vi "niTuner Get Cal (multi).vi"(8 "error in":errorcluster, 9 "correct for attenuation":bool=TRUE, 11 "taskID in":i32 format="%.0x") -> (0 "error out":errorcluster, 2 "calibrations":T1(array[cluster]) {"array" format="%.2f"; "f2" format="%.2f"; "f1" format="%.2f"}, 3 "taskID out":i32 format="%.0x")   [LabVIEW 2011]
doc: "This polymorph returns calibration information for multiple frequency entries in the scan list. Each frequency entry returns an RF calibration coefficient, an IF calibration coefficient, and (if include attenuation is set to TRUE) a total attenuation calibration coefficient."
uses:
  nipxi5600u.dll
  nidaq32.dll
panel:
  out "RF tuned frequencies":dbl[](graph)
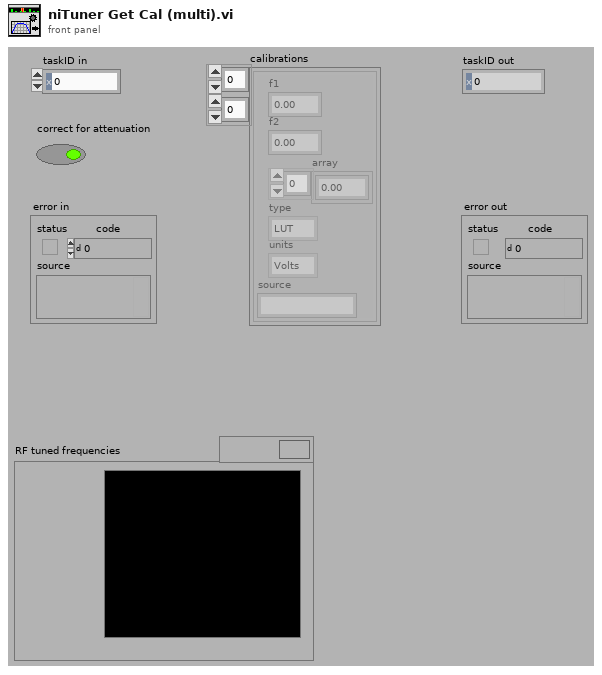
[diagram p1: front panel]
types:
  T1 = cluster{"f1":dbl, "f2":dbl, "array":sgl[], "type":enum16{"LUT", "polynomial"}, "units":enum16{"Volts", "Watts", "dBm", "dBW", "dBV", "dBmV", "dBuV"}, "source":string}[][]
  T2 = cluster{"f1":dbl, "f2":dbl, "array":sgl[], "type":enum16{"LUT", "polynomial"}, "units":enum16{"Volts", "Watts", "dBm", "dBW", "dBV", "dBmV", "dBuV"}, "source":string}
  T3 = cluster{"f1":dbl, "f2":dbl, "array":sgl[], "type":enum16{"LUT", "polynomial"}, "units":enum16{"Volts", "Watts", "dBm", "dBW", "dBV", "dBmV", "dBuV"}, "source":string}[]
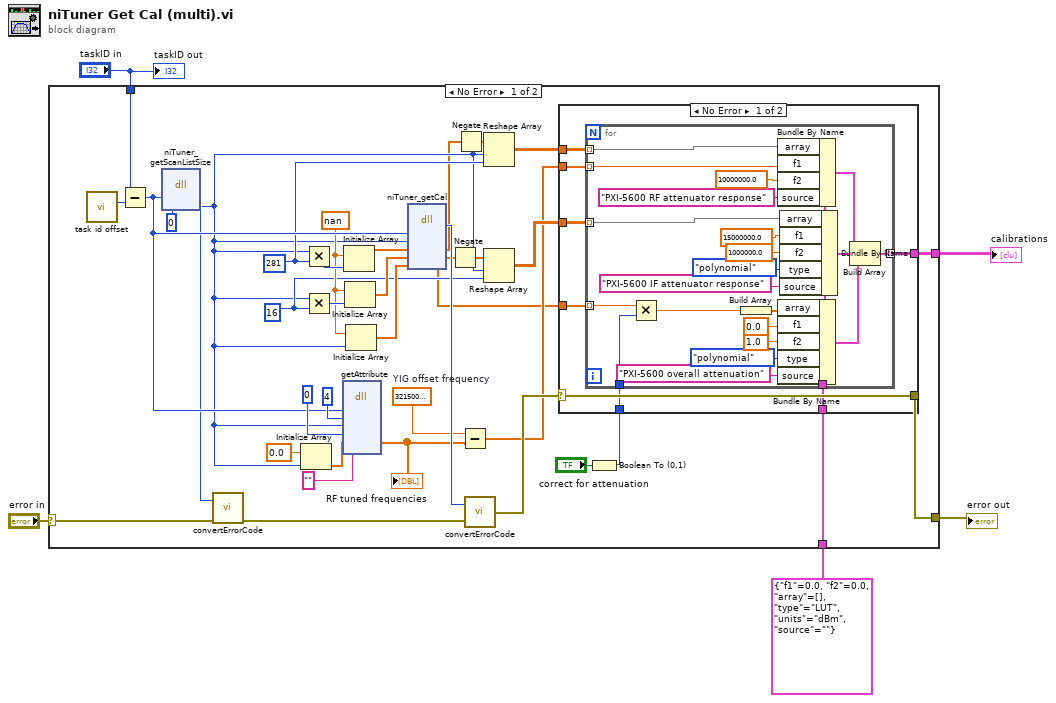
[diagram p0: block diagram]
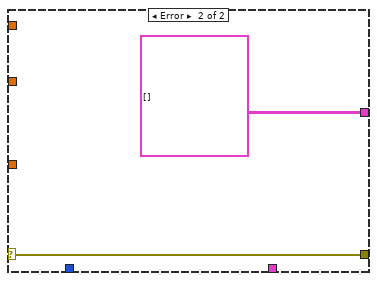
[diagram p2: hidden frame]
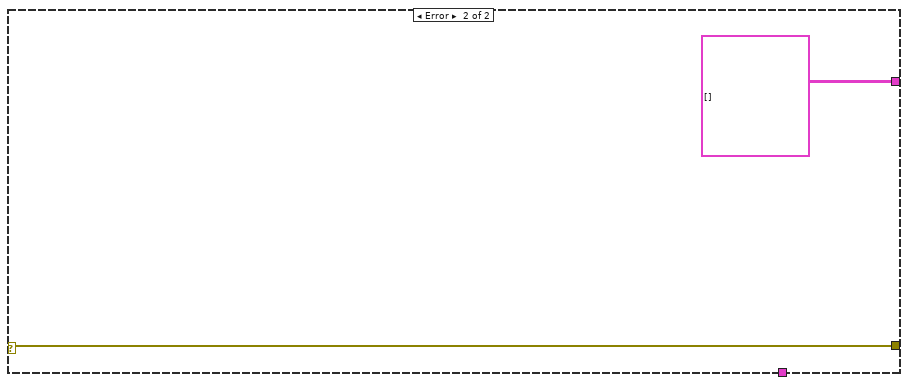
[diagram p3: hidden frame]
diagram:
  n1 = case shown="No Error" "error in" {
    selector: "error in" -> [w23 w77]
    tunnel: T2 {"f1"=0.0, "f2"=0.0, "array"=[], "type"=enum."LUT", "units"=enum."dBm", "source"=""} -> [w41 _]
    tunnel: [w40 w77] -> w3
    tunnel: "taskID in" -> [w39 _]
    tunnel: [w14 T1 []] -> w1
    frame No Error {
      w16 = 3215000000.0  # YIG offset frequency
      w27 = nan ("Element Data")
      w19 = u32 16
      w20 = u32 281
      n2 = call <instrlib>:"task id offset.vi"() -> ("taskID offset"=w43:i32)
      n3 = Subtract(x=w39, y=w43) -> (x-y=w31:i32)
      n4 = dll-call lib="nipxi5600u.dll" fn="niTuner_getScanListSize"("taskID"=w31, "scanListSize"=u32 0) -> (w24:i32, "scanListSize"=w11:u32)  [unwired: 4 in, 2 out]
      n5 = call <instrlib>:"convertErrorCode.vi"("error in"=w23, "error code"=w24) -> ("error out"=w22:errorcluster)
      n6 = Initialize Array(0.0 ("Element Data"), w11) -> (w36:dbl[])
      n7 = Multiply(x=w11, y=w20) -> (x*y=w29:u32)
      n8 = Multiply(x=w11, y=w19) -> (x*y=w28:u32)
      n9 = dll-call lib="nidaq32.dll" fn="getAttribute"("device"=w31, "attribute"=u32 4, "u32val"=w11, "i32val"=0, "f64val"=w36, "strval"="") -> ("f64val"=w17:dbl[])  [unwired: 9 in, 2 out]
      "RF tuned frequencies" <- w17
      n10 = Initialize Array(w27, w29) -> (w30:dbl[])
      n11 = Initialize Array(w27, w28) -> (w26:dbl[])
      n12 = Initialize Array(w27, w11) -> (w25:dbl[])
      n13 = dll-call lib="nipxi5600u.dll" fn="niTuner_getCal"("taskID"=w31, "listSize"=w11, "RFArrays"=w30, "IFArrays"=w26, "attenuationArray"=w25) -> (w42:i32, "RFArrays"=w9:dbl[], "IFArrays"=w8:dbl[], "attenuationArray"=w10:dbl[])  [unwired: 5 in, 2 out]
      n14 = Negate(x=w8) -> (-x=w6:dbl[])
      n15 = Negate(x=w9) -> (-x=w7:dbl[])
      n16 = Subtract(x=w16, y=w17) -> (x-y=w15:dbl[])
      n17 = call <instrlib>:"convertErrorCode.vi"("error in"=w22, "error code"=w42) -> ("error out"=w21:errorcluster)
      n18 = Reshape Array(w7, w11, w20) -> (w38:dbl[][])
      n19 = Reshape Array(w6, w11, w19) -> (w18:dbl[][])
      n20 = Boolean To (0,1)(Boolean="correct for attenuation") -> (0, 1=w12:i16)
      n21 = case shown="No Error" w21 {
        selector: w21 -> [w50 w75]
        tunnel: w38 -> [w51 _]
        tunnel: w41 -> [w46 _]
        tunnel: [w50 w75] -> w40
        tunnel: w15 -> [w49 _]
        tunnel: w18 -> [w48 _]
        tunnel: w10 -> [w47 _]
        tunnel: [w45 T1 []] -> w14
        tunnel: w12 -> [w44 _]
        frame No Error {
          n22 = for {
            tunnel: w51 -> [w73] mode=indexing
            tunnel: w49 -> [w70] mode=indexing
            tunnel: w48 -> [w69] mode=indexing
            tunnel: w47 -> [w62] mode=indexing
            tunnel: w46 -> [w64]
            tunnel: [w54] -> w45 mode=indexing
            tunnel: w44 -> [w52]
            n23 = Multiply(x=w62, y=w52) -> (x*y=w53:dbl)
            n24 = Build Array(w53) -> (w63:dbl[])
            n25 = Bundle By Name(cluster=w64, "array"=w73, "f1"=w70, "f2"=10000000.0, "source"="PXI-5600 RF attenuator response") -> (w57:T2)
            n26 = Bundle By Name(cluster=w64, "array"=w63, "f1"=0.0, "f2"=1.0, "type"=enum16{"LUT", "polynomial"}."polynomial", "source"="PXI-5600 overall attenuation") -> (w56:T2)
            n27 = Bundle By Name(cluster=w64, "array"=w69, "f1"=15000000.0, "f2"=1000000.0, "type"=enum16{"LUT", "polynomial"}."polynomial", "source"="PXI-5600 IF attenuator response") -> (w58:T2)
            n28 = Build Array(w57, w58, w56) -> (w54:T3)
          }
        }
        frame Error {
        }
      }
    }
    frame Error {
    }
  }
  "calibrations" <- w1
  "error out" <- w3
  "taskID out" <- "taskID in"
